vi "util_get_change_out.vi"(7 "references":T1, 8 "error in (no error)":errorcluster, 10 "timeout":i32) -> (0 "error out":errorcluster, 2 "data":variant, 3 "change?":bool)   [LabVIEW 2015, in "repub-dvr_nre.lvlib"]
uses:
  repub-dvr_nre.lvlib
  _controls/references.ctl
  private/_controls/input.ctl
  private/_controls/input_command.ctl
  private/_controls/output.ctl
  private/_controls/data.ctl
  _controls/configuration.ctl
  lv-recipe-machine/private/_controls/recipe_data.ctl
  lv-recipe-machine/public/_controls/mode.ctl
  lv-recipe-machine/public/_controls/manual_state.ctl
  lv-recipe-machine/public/_controls/automatic_state.ctl
  <userlib>/antonio-alexander/lv-waitgroup/public/_controls/api_waitgroup.ctl
  lv-recipe-machine/public/_controls/transition.ctl
  _controls/change.ctl
  lv-recipe-machine/lv-recipe-machine.lvlib
  <userlib>/antonio-alexander/lv-waitgroup/lv-waitgroup.lvlib
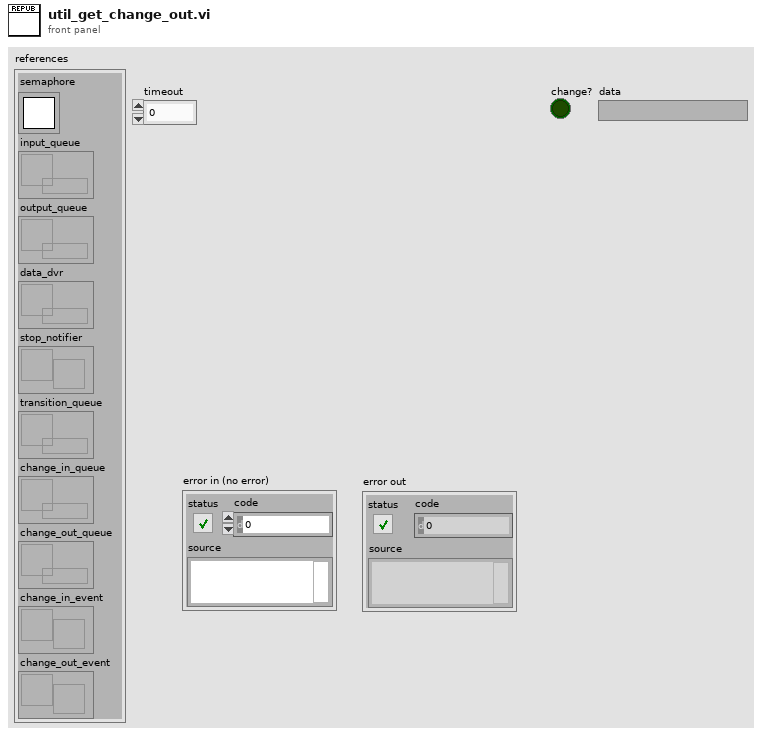
[diagram p1: front panel]
types:
  T1 = typedef "repub-dvr_nre.lvlib/references.ctl" = cluster{"semaphore":T2, "input_queue":refnum<queue>, "output_queue":refnum<queue>, "data_dvr":refnum<data-value>, "stop_notifier":refnum<notifier>, "transition_queue":refnum<queue>, "change_in_queue":refnum<queue>, "change_out_queue":refnum<queue>, "change_in_event":refnum<user-event>, "change_out_event":refnum<user-event>}
  T2 = typedef "Semaphore RefNum" = refnum<k1>
  T3 = typedef "repub-dvr_nre.lvlib/change.ctl" = cluster{"changed":bool, "data":variant}
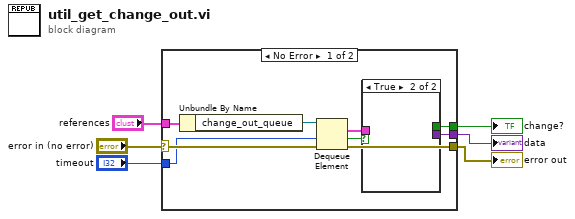
[diagram p0: block diagram]
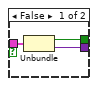
[diagram p2: hidden frame]
diagram:
  n1 = case shown="No Error" "error in (no error)" {
    selector: "error in (no error)" -> [w8 w19]
    tunnel: [w13 w19] -> w5
    tunnel: "references" -> [w15 _]
    tunnel: "timeout" -> [w7 _]
    tunnel: [w10 _] -> w2
    tunnel: [w9 _] -> w1
    frame No Error {
      n2 = Unbundle By Name(w15) -> ("change_out_queue"=w14:refnum<queue>)
      n3 = Dequeue Element(queue=w14, timeout in ms (-1)=w7, error in (no error)=w8) -> (element=w11:T3, timed out?=w12:bool, error out=w13:errorcluster)  [unwired: 1 out]
      n4 = case shown="True" w12 {
        tunnel: w11 -> [w18 _]
        tunnel: [w17 _] -> w10
        tunnel: [w16 _] -> w9
        frame False {
          n5 = Unbundle(w18) -> ("changed"=w17:bool, "data"=w16:variant)
        }
        frame True {
        }
      }
    }
    frame Error {
    }
  }
  "error out" <- w5
  "change?" <- w2
  "data" <- w1
